vi "OPC.vi"() -> ()   [LabVIEW 2018]
uses:
  C:/Users/gpour/source/repos/LibUA/NET/LibUA/bin/Release/LibUA.dll
  source/repos/LibUA/NET/LibUA/bin/Release/LibUA.dll
panel:
  in  "value":string
  in  "index":u32
  out "test 2":string
  in  "Set Values":u32
  in  "SetValue":string
  out "Getvalue":string
  in  "GetValues":u32
  in  "test":bool
  in  "Lire":bool
  in  "Ecrire":bool
  in  "cheminconf":string="C:\\Users\\gpour\\source\\repos\\LibUA\\NET\\LibUA\\bin\\Release\\cfg.ini"
  in  "port":i32=7718
  in  "appname":string="OPTEC-WithinLV"
  out "TestServer":refnum<k24>
  in  "Quit":bool
  in  "Stop Serv":bool
  in  "Start Serv":bool
  # "SET VALUES"
  # "GET VALUES"
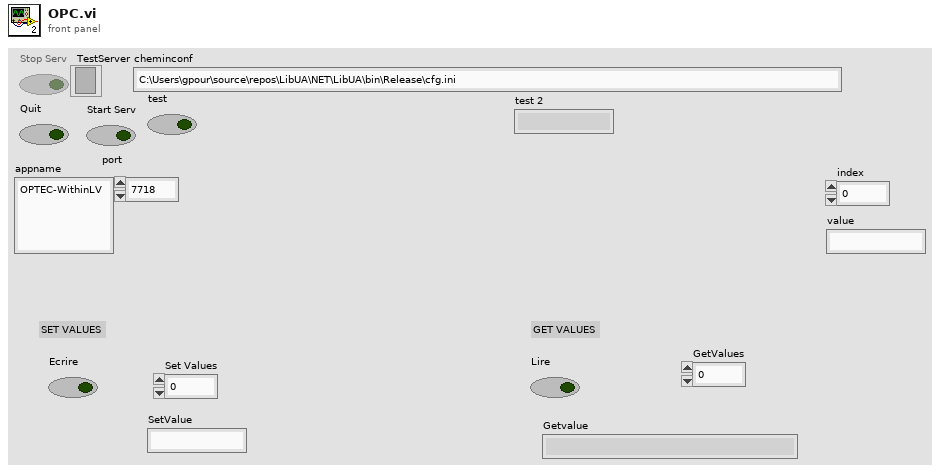
[diagram p1: front panel]
types:
  T1 = enum8{"Enabled", "Disabled", "Disabled and Grayed Out"}
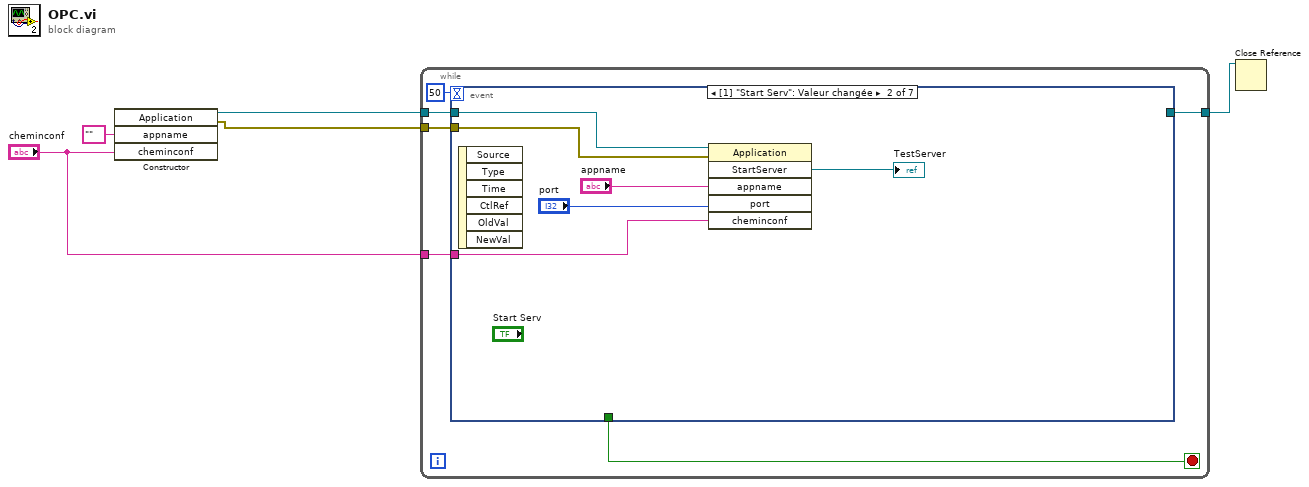
[diagram p0: block diagram]
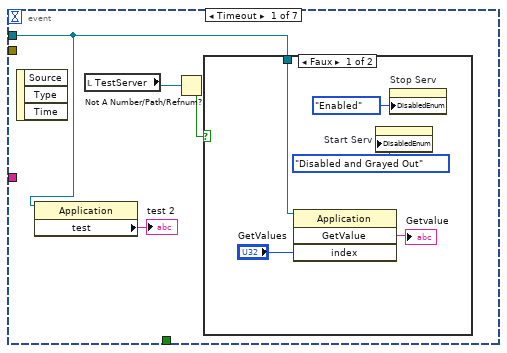
[diagram p2: hidden frame]
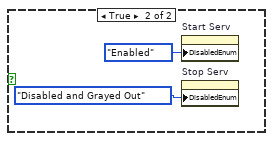
[diagram p3: hidden frame]
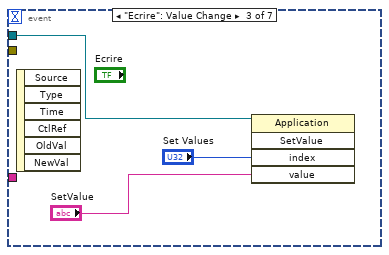
[diagram p4: hidden frame]
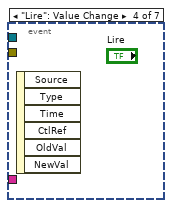
[diagram p5: hidden frame]
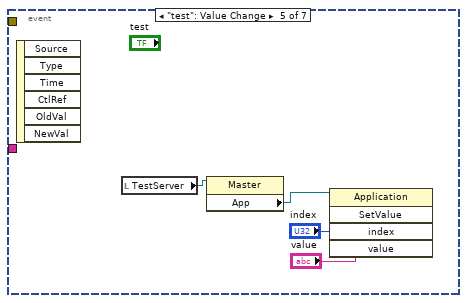
[diagram p6: hidden frame]
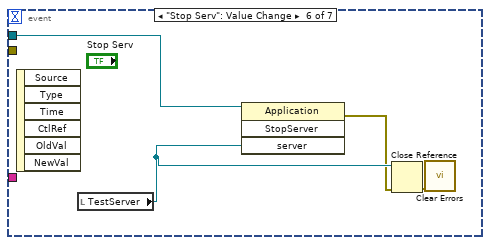
[diagram p7: hidden frame]
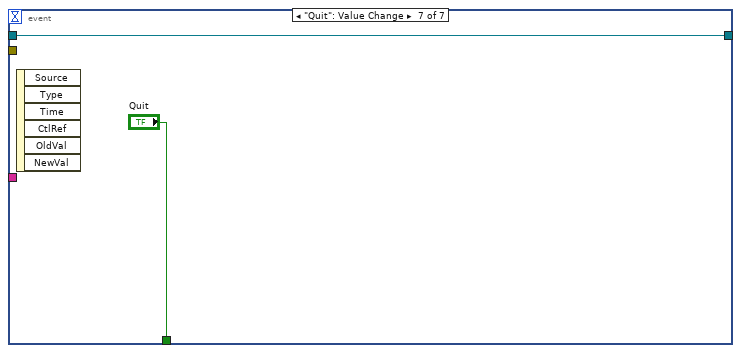
[diagram p8: hidden frame]
diagram:
  n1 = constructor class="Application"("appname"="", "cheminconf"="cheminconf") -> (reference out=w5:refnum<k24>, error out=w4:errorcluster)  [unwired: 3 in, 3 out]
  n2 = while {
    tunnel: w5 -> [w11]
    tunnel: w4 -> [w10]
    tunnel: [w8] -> w2
    tunnel: "cheminconf" -> [w7]
    stop <- w9 stop-if-true
    n3 = event shown="[1] \"Start Serv\": Valeur changée" {
      selector: _ -> [_ _ _ _ _ _ _]
      dyn-events: _ -> [_ _ _ _ _ _ _]
      timeout: 50 -> [_ _ _ _ _ _ _]
      tunnel: w11 -> [w13 w28 w31 _ _ w39 w40]
      tunnel: w10 -> [_ w27 _ _ _ _ _]
      tunnel: [_ _ _ _ _ _ "Quit"] -> w9
      tunnel: [_ _ _ _ _ _ w40] -> w8
      tunnel: w7 -> [_ w23 _ _ _ _ _]
      event Timeout {
        n4 = event-data() -> ()  [unwired: 1 in, 3 out]
        n5 = property class="Application"(reference=w13) -> ("test"=→"test 2":string)  [unwired: 1 in, 2 out]
        n6 = local read "TestServer"() -> (w15:refnum<k24>)
        n7 = Not A Number/Path/Refnum?(number/path/refnum=w15) -> (NaN/Path/Refnum?=w14:bool)
        n8 = case shown="Faux" w14 {
          tunnel: w13 -> [w17 _]
          frame False {
            n9 = invoke on="Nœud de méthode" class="Application" method="GetValue"(reference=w17, "index"="GetValues") -> ("GetValue"=→"Getvalue":string)  [unwired: 2 in, 3 out]
            n10 = property on="Start Serv" class="Bool"("DisabledEnum"=T1."Disabled and Grayed Out" ("Désactivé")) -> ()  [unwired: 2 in, 2 out]
            n11 = property on="Stop Serv" class="Bool"("DisabledEnum"=T1."Enabled" ("Désactivé")) -> ()  [unwired: 2 in, 2 out]
          }
          frame True {
            n12 = property on="Start Serv" class="Bool"("DisabledEnum"=T1."Enabled" ("Désactivé")) -> ()  [unwired: 2 in, 2 out]
            n13 = property on="Stop Serv" class="Bool"("DisabledEnum"=T1."Disabled and Grayed Out" ("Désactivé")) -> ()  [unwired: 2 in, 2 out]
          }
        }
      }
      event "Start Serv": Value Change {
        n14 = event-data() -> ()  [unwired: 1 in, 6 out]
        n15 = invoke class="Application" method="StartServer"(reference=w28, error in=w27, "appname"="appname", "port"="port", "cheminconf"=w23) -> ("StartServer"=→"TestServer":refnum<k24>)  [unwired: 1 in, 5 out]
      }
      event "Ecrire": Value Change {
        n16 = event-data() -> ()  [unwired: 1 in, 6 out]
        n17 = invoke class="Application" method="SetValue"(reference=w31, "index"="Set Values", "value"="SetValue") -> ()  [unwired: 2 in, 5 out]
      }
      event "Lire": Value Change {
        n18 = event-data() -> ()  [unwired: 1 in, 6 out]
      }
      event "test": Value Change {
        n19 = event-data() -> ()  [unwired: 1 in, 6 out]
        n20 = local read "TestServer"() -> (w35:refnum<k24>)
        n21 = property class="Master"(reference=w35) -> ("App"=w32:refnum<k24>)  [unwired: 1 in, 2 out]
        n22 = invoke class="Application" method="SetValue"(reference=w32, "index"="index", "value"="value") -> ()  [unwired: 2 in, 5 out]
      }
      event "Stop Serv": Value Change {
        n23 = event-data() -> ()  [unwired: 1 in, 6 out]
        n24 = local read "TestServer"() -> (w38:refnum<k24>)
        n25 = invoke class="Application" method="StopServer"(reference=w39, "server"=w38) -> (error out=w37:errorcluster)  [unwired: 2 in, 3 out]
        n26 = Close Reference(reference=w38, error in (no error)=w37) -> (error out=w36:errorcluster)
        n27 = call <vilib>:"Clear Errors.vi"("error in (no error)"=w36) -> ()  [unwired: 5 in, 2 out]
      }
      event "Quit": Value Change {
        n28 = event-data() -> ()  [unwired: 1 in, 6 out]
      }
    }
  }
  n29 = Close Reference(reference=w2) -> ()  [unwired: 1 in, 1 out]
